vi "Dequeue.vi"(8 "error in (no error)":errorcluster, 11 "MASTER in":refnum<class "MASTER.lvclass">) -> (0 "error out":errorcluster, 3 "MASTER out":refnum<class "MASTER.lvclass">, 6 "state":string)   [LabVIEW 2014, in "Files Library.lvlib" / "Master.lvclass"]
uses:
  MASTER/MASTER.lvclass
  MASTER/MASTER.lvclass/MASTER.ctl
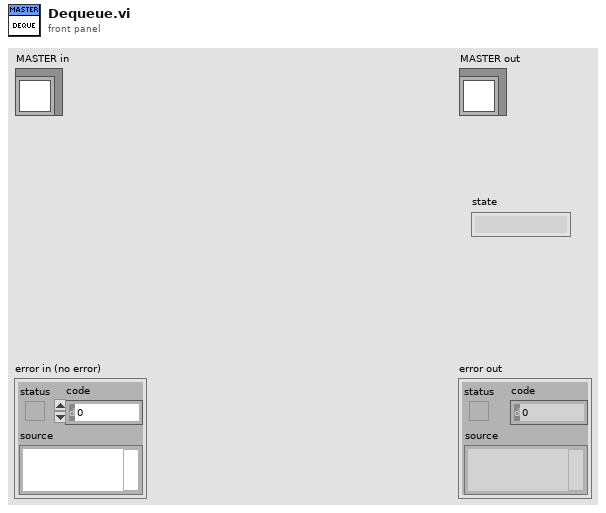
[diagram p1: front panel]
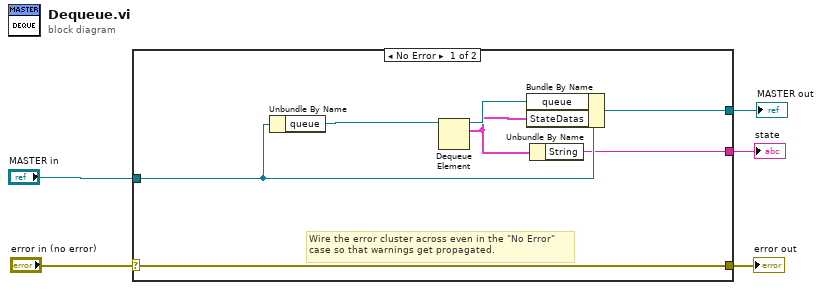
[diagram p0: block diagram]
diagram:
  n1 = case shown="No Error" "error in (no error)" {
    selector: "error in (no error)" -> [w12 w14]
    tunnel: [w12 w14] -> w4
    tunnel: [w8 w13] -> w2
    tunnel: "MASTER in" -> [w9 w13]
    tunnel: [w6 _] -> w1
    frame No Error {
      # "Wire the error cluster across even in the \"No Error\"\ncase so that warnings get propagated."
      n2 = Unbundle By Name(w9) -> ("queue"=w11:refnum<queue>)
      n3 = Dequeue Element(queue=w11) -> (queue out=w10:refnum<queue>, element=w7:cluster{"String":string, "Data":variant})  [unwired: 2 in, 2 out]
      n4 = Bundle By Name(cluster=w9, "queue"=w10, "StateDatas"=w7) -> (w8:refnum<class "MASTER.lvclass">)
      n5 = Unbundle By Name(w7) -> ("String"=w6:string)
    }
    frame Error {
    }
  }
  "error out" <- w4
  "MASTER out" <- w2
  "state" <- w1
